vi "Parse.vi"(8 "Error In":errorcluster, 11 "Parser In":refnum<class "Parser.lvclass">) -> (0 "Error Out":errorcluster, 2 "Tokens":refnum<class "Abstract.lvclass">[](array[class]), 3 "Parser Out":refnum<class "Parser.lvclass">)   [LabVIEW 2017, in "Mustache.lvlib" / "Parser.lvclass"]
uses:
  Parser.lvclass
  Tokens/Public/Abstract/Abstract.lvclass
  Parser.lvclass/Parser.ctl
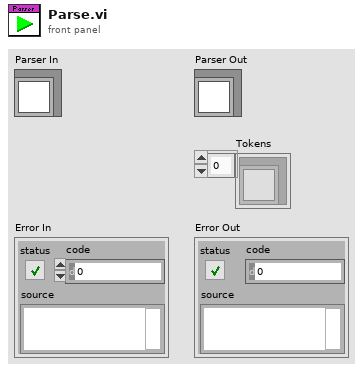
[diagram p1: front panel]
types:
  T1 = typedef "Mustache.lvlib/Parser.lvclass/States.ctl" = enum16{"Text", "Open Delimiter", "Tag", "Close Delimiter"}
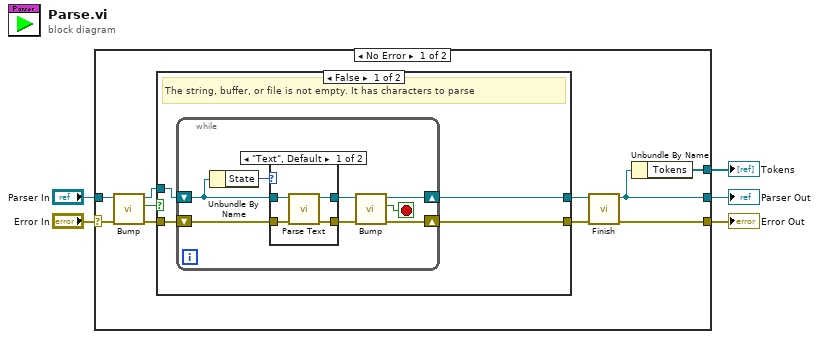
[diagram p0: block diagram]
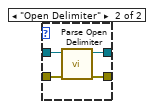
[diagram p2: hidden frame]
diagram:
  n1 = case shown="No Error" "Error In" {
    selector: "Error In" -> [w13 w39]
    tunnel: "Parser In" -> [w12 w38]
    tunnel: [w6 w39] -> w3
    tunnel: [w8 w38] -> w2
    tunnel: [w14 _] -> w1
    frame No Error {
      n2 = call "Bump.vi"("Error In"=w13, "Parser In"=w12) -> ("Error Out"=w10:errorcluster, "Done"=w9:bool, "Parser Out"=w11:refnum<class "Parser.lvclass">)  [unwired: 7 in]
      n3 = case shown="False" w9 {
        tunnel: [w17 w36] -> w7
        tunnel: [w16 w37] -> w15
        tunnel: w10 -> [w19 w36]
        tunnel: w11 -> [w18 w37]
        frame False {
          # "The string, buffer, or file is not empty. It has characters to parse"
          n4 = while {
            shift-right: [w21] -> w17
            shift-left: w19 -> [w25]
            shift-right: [w23] -> w16
            shift-left: w18 -> [w26]
            stop <- w22 stop-if-true
            n5 = Unbundle By Name(w26) -> ("State"=w27:T1)
            n6 = case shown="\"Text\", Default" w27 {
              tunnel: w25 -> [w30 w35]
              tunnel: w26 -> [w31 w34]
              tunnel: [w29 w33] -> w24
              tunnel: [w28 w32] -> w20
              frame "Text", Default {
                n7 = call "Parse Text.vi"("Error In"=w30, "Parser In"=w31) -> ("Error Out"=w28:errorcluster, "Parser Out"=w29:refnum<class "Parser.lvclass">)  [unwired: 8 in]
              }
              frame "Open Delimiter" {
                n8 = call "Parse Open Delimiter.vi"("Error In"=w35, "Parser In"=w34) -> ("Error Out"=w32:errorcluster, "Parser Out"=w33:refnum<class "Parser.lvclass">)  [unwired: 8 in]
              }
            }
            n9 = call "Bump.vi"("Error In"=w20, "Parser In"=w24) -> ("Error Out"=w21:errorcluster, "Done"=w22:bool, "Parser Out"=w23:refnum<class "Parser.lvclass">)  [unwired: 7 in]
          }
        }
        frame True {
          # "The string, buffer, file, etc. is empty. There is nothing to do."
        }
      }
      n10 = call "Finish.vi"("Error In"=w7, "Parser In"=w15) -> ("Error Out"=w6:errorcluster, "Parser Out"=w8:refnum<class "Parser.lvclass">)  [unwired: 8 in]
      n11 = Unbundle By Name(w8) -> ("Tokens"=w14:refnum<class "Abstract.lvclass">[])
    }
    frame Error {
    }
  }
  "Error Out" <- w3
  "Parser Out" <- w2
  "Tokens" <- w1
